vi "Up Sample Plot - TOI.vi"(10 "add N sample between points":i32, 11 "Plot":dbl[](array[numeric])) -> (3 "Ramp Pattern":dbl[](array[numeric]))   [LabVIEW 2023]
uses:
  <vilib>/Analysis/1siggen.llb/Ramp Pattern by Samples.vi
  <vilib>/Analysis/NI_AALBase.lvlib
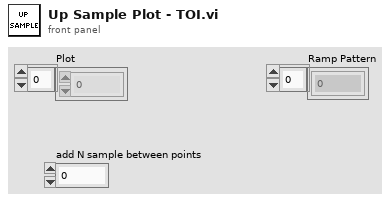
[diagram p1: front panel]
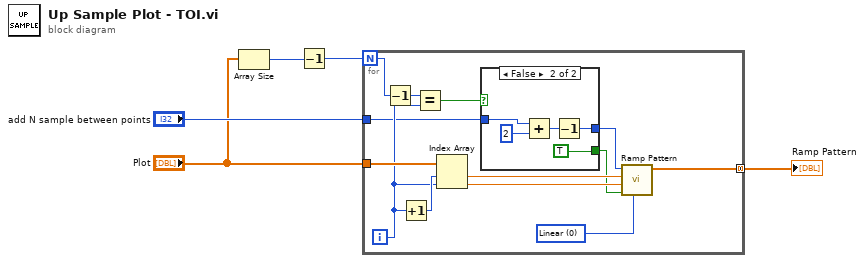
[diagram p0: block diagram]
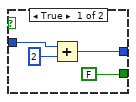
[diagram p2: hidden frame]
diagram:
  n1 = Array Size(array="Plot") -> (size(s)=w3:i32)
  n2 = Decrement(x=w3) -> (x-1=w4:i32)
  n3 = for {
    N: w4 -> [w14]
    tunnel: "Plot" -> [w18]
    tunnel: [w12] -> w2 mode=concatenating
    tunnel: "add N sample between points" -> [w7]
    i -> [w8]
    w6 = u16 0 items=["Linear", "Logarithmic"] ("type")
    n4 = Decrement(x=w14) -> (x-1=w13:i32)
    n5 = Increment(x=w8) -> (x+1=w17:i32)
    n6 = Equal?(x=w13, y=w8) -> (x = y?=w11:bool)
    n7 = Index Array(array=w18, index #1=w17, index #2=w8) -> (element #1=w16:dbl, element #2=w15:dbl)
    n8 = case shown="False" w11 {
      tunnel: [FALSE TRUE] -> w10
      tunnel: [w20 w24] -> w9
      tunnel: w7 -> [w19 w23]
      frame True {
        n9 = Add(x=w19, y=2) -> (x+y=w20:i32)
      }
      frame False {
        n10 = Add(x=w23, y=2) -> (x+y=w25:i32)
        n11 = Decrement(x=w25) -> (x-1=w24:i32)
      }
    }
    n12 = call-poly <vilib>:"Ramp Pattern.vi"("type"=w6, "exclude end?"=w10, "start"=w15, "end"=w16, "samples"=w9) -> ("Ramp Pattern"=w12:dbl[])  [unwired: 5 in, 1 out]
  }
  "Ramp Pattern" <- w2
